vi "GetType.vi"(8 "error in (no error)":errorcluster, 11 "Initiate Msg":refnum<class "Initiate Msg.lvclass">) -> (0 "error out":errorcluster, 2 "Data Sample":variant, 3 "Initiate Msg":refnum<class "Initiate Msg.lvclass">)   [LabVIEW 2015, in "CS++DMM.lvlib" / "Initiate Msg.lvclass"]
uses:
  Initiate Msg.lvclass
  Initiate Msg.lvclass/Initiate Msg.ctl
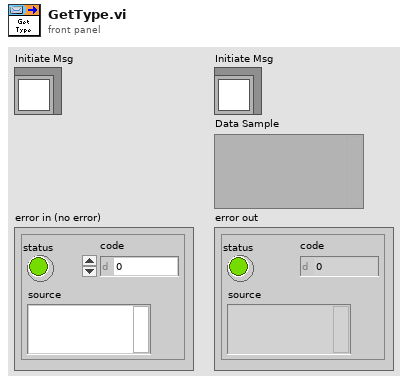
[diagram p1: front panel]
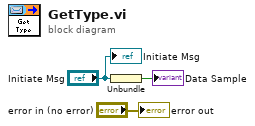
[diagram p0: block diagram]
diagram:
  n1 = Unbundle("Initiate Msg") -> (→"Data Sample":bool)
  "error out" <- "error in (no error)"
  "Initiate Msg" <- "Initiate Msg"
